vi "EnemyKick.vi"(6 "atacando contra?":bool, 9 "balls":T1[](array[typedef]), 10 "Field Size in":T5, 11 "Robot in":T2={"id"=0, "function"=enum."Attacker", "x"=0.0, "y"=0.0, "orientation"=0.0, "v_tangent"=0.0, "v_normal"=0.0, "v_ang"=0.0, "kick_x"=0.0, "kick_z"=0.0, "dribble"=FALSE, "Timestamp"=timestamp(0 s since 1904-01-01), "dest_x"=0.0, "dest_y"=0.0, "dest_orientation"=0.0, "estimatives"={"est_v_tangent"=0.0, "est_v_normal"=0.0, "est_vx"=0.0, "est_vy"=0.0, "Pos Robot Est"=[]}, "dest_x_kick"=0.0, "dest_y_kick"=0.0, "Gap Coord"=[], "States"=enum."GoToTangent"}) -> (3 "Robot out":T2={"id"=0, "function"=enum."Attacker", "x"=0.0, "y"=0.0, "orientation"=0.0, "v_tangent"=0.0, "v_normal"=0.0, "v_ang"=0.0, "kick_x"=0.0, "kick_z"=0.0, "dribble"=FALSE, "Timestamp"=timestamp(0 s since 1904-01-01), "dest_x"=0.0, "dest_y"=0.0, "dest_orientation"=0.0, "estimatives"={"est_v_tangent"=0.0, "est_v_normal"=0.0, "est_vx"=0.0, "est_vy"=0.0, "Pos Robot Est"=[]}, "dest_x_kick"=0.0, "dest_y_kick"=0.0, "Gap Coord"=[], "States"=enum."GoToTangent"})   [LabVIEW 2017]
uses:
  Core/Field Size.ctl
  Core/AI Robot.ctl
  Functions Enum.ctl
  AttackerStates.ctl
  Core/AI Ball.ctl
  <vilib>/Analysis/_algsub.llb/Real Vector Norm.vi
  <vilib>/Analysis/NI_AALPro.lvlib
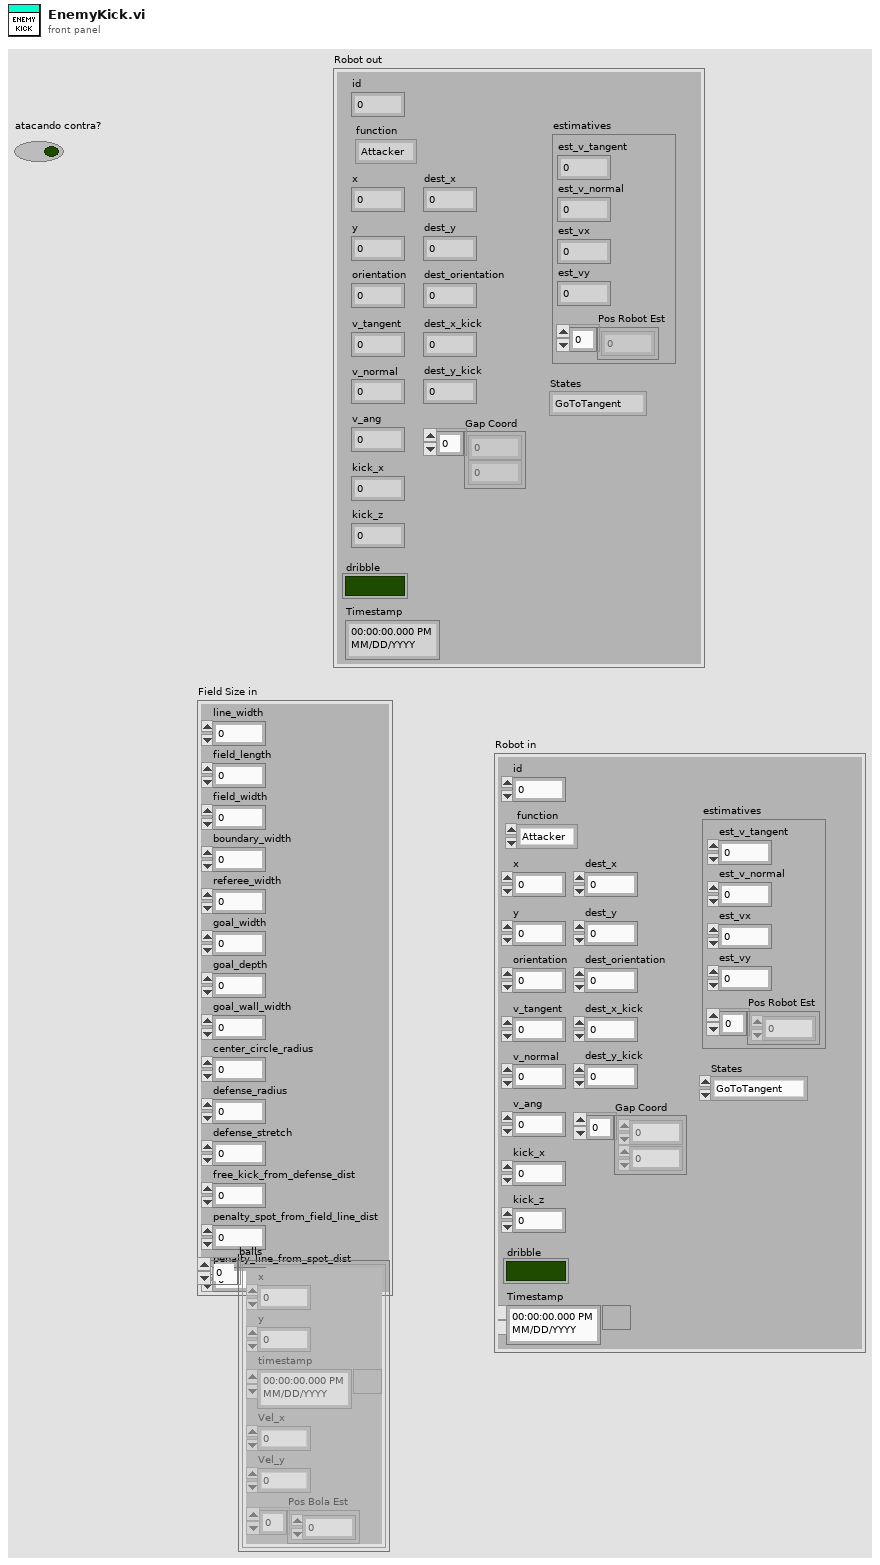
[diagram p1: front panel]
types:
  T1 = typedef "AI Ball.ctl" = cluster{"x":dbl, "y":dbl, "timestamp":timestamp, "Vel_x":dbl, "Vel_y":dbl, "Pos Bola Est":dbl[]}
  T2 = typedef "AI Robot.ctl" = cluster{"id":u32, "function":T3, "x":dbl, "y":dbl, "orientation":dbl, "v_tangent":dbl, "v_normal":dbl, "v_ang":dbl, "kick_x":dbl, "kick_z":dbl, "dribble":bool, "Timestamp":timestamp, "dest_x":dbl, "dest_y":dbl, "dest_orientation":dbl, "estimatives":cluster{"est_v_tangent":dbl, "est_v_normal":dbl, "est_vx":dbl, "est_vy":dbl, "Pos Robot Est":dbl[]}, "dest_x_kick":dbl, "dest_y_kick":dbl, "Gap Coord":dbl[], "States":T4}
  T3 = typedef "Functions Enum.ctl" = enum16{"Attacker", "Goalie", "Defender", "Striker", "Goto 0", "Dummy", "Kicker", "ZigZag"}
  T4 = typedef "AttackerStates.ctl" = enum16{"Pass", "GoToTangent", "BallGetting", "GoToKick", ""}
  T5 = typedef "Field Size.ctl" = cluster{"line_width":u32, "field_length":u32, "field_width":u32, "boundary_width":u32, "referee_width":u32, "goal_width":u32, "goal_depth":u32, "goal_wall_width":u32, "center_circle_radius":u32, "defense_radius":u32, "defense_stretch":u32, "free_kick_from_defense_dist":u32, "penalty_spot_from_field_line_dist":u32, "penalty_line_from_spot_dist":u32}
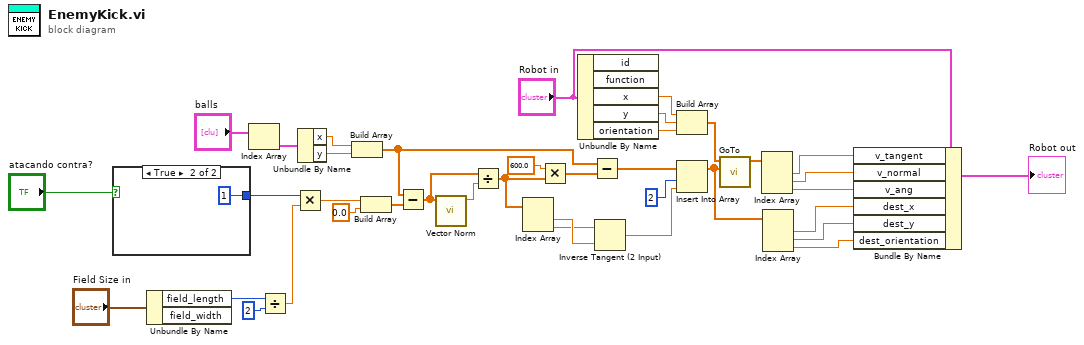
[diagram p0: block diagram]
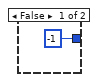
[diagram p2: hidden frame]
diagram:
  n1 = case shown="True" "atacando contra?" {
    tunnel: [-1 1] -> w18
    frame False {
    }
    frame True {
    }
  }
  n2 = Unbundle By Name("Field Size in") -> ("field_length"=w37:u32)  [unwired: 1 out]
  n3 = Index Array(array="balls") -> (element=w33:T1)  [unwired: 1 in]
  n4 = Divide(x=w37, y=u32 2) -> (x/y=w28:dbl)
  n5 = Multiply(x=w18, y=w28) -> (x*y=w17:dbl)
  n6 = Unbundle By Name(w33) -> ("x"=w35:dbl, "y"=w34:dbl)
  n7 = Build Array(w35, w34) -> (w19:dbl[])
  n8 = Build Array(w17, 0.0 ("element")) -> (w13:dbl[])
  n9 = Subtract(x=w19, y=w13) -> (x-y=w14:dbl[])
  n10 = call-poly <vilib>:"Vector Norm.vi"("Input Vector"=w14) -> ("norm"=w15:dbl)  [unwired: 9 in, 1 out]
  n11 = Divide(x=w14, y=w15) -> (x/y=w8:dbl[])
  n12 = Index Array(array=w8) -> (element #1=w10:dbl, element #2=w9:dbl)  [unwired: 2 in]
  n13 = Multiply(x=600.0, y=w8) -> (x*y=w6:dbl[])
  n14 = Unbundle By Name("Robot in") -> ("x"=w32:dbl, "y"=w31:dbl, "orientation"=w30:dbl)  [unwired: 2 out]
  n15 = Subtract(x=w19, y=w6) -> (x-y=w5:dbl[])
  n16 = Inverse Tangent (2 Input)(1:w10, 2:w9) -> (0:w11:dbl)
  n17 = Build Array(w32, w31, w30) -> (w20:dbl[])
  n18 = Insert Into Array(array=w5, index=2, new element=w11) -> (w4:dbl[])
  n19 = call "GoTo.vi"("Target"=w4, "Position"=w20) -> ("Output\nVelocity"=w22:dbl[])  [unwired: 8 in, 1 out]
  n20 = Index Array(array=w22) -> (element #1=w25:dbl, element #2=w26:dbl, element #3=w27:dbl)  [unwired: 3 in]
  n21 = Index Array(array=w4) -> (element #1=w3:dbl, element #2=w2:dbl, element #3=w1:dbl)  [unwired: 3 in]
  n22 = Bundle By Name(cluster="Robot in", "v_tangent"=w25, "v_normal"=w26, "v_ang"=w27, "dest_x"=w3, "dest_y"=w2, "dest_orientation"=w1) -> (→"Robot out":T2)
